vi "file control.vi"(7 "para3":u32, 8 "error in (no error)":errorcluster, 9 "op":i32, 10 "zDbName":string, 11 "para0":dbl) -> (0 "error out":errorcluster, 2 "function return":i32, 3 "para0 out":dbl, 5 "para3 out":u32)   [LabVIEW 2020, in "sqlite3.lvlib"]
uses:
  sqlite3.lvlib
  errstr.vi
  bin/sqlite3_64.dll
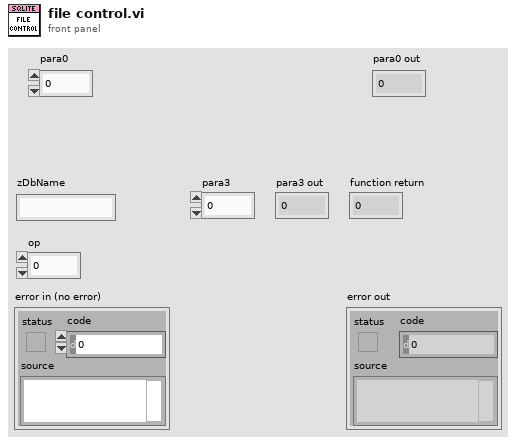
[diagram p1: front panel]
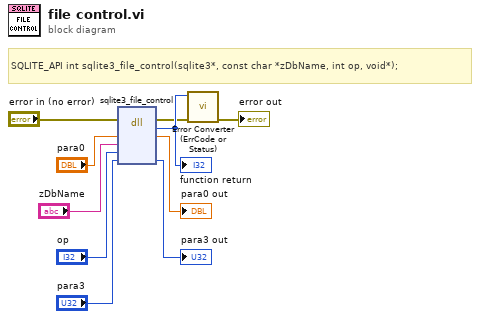
[diagram p0: block diagram]
diagram:
  # "SQLITE_API int sqlite3_file_control(sqlite3*, const char *zDbName, int op, void*);"
  n1 = dll-call lib="C:/Users/Fred.Guo/Desktop/Database-configuration/externals/sqlite3/Source/bin/sqlite3_*.*" fn="sqlite3_file_control"(error in="error in (no error)", "para0"="para0", "zDbName"="zDbName", "op"="op", "para3"="para3") -> (error out=w2:errorcluster, w10:i32, "para0"=→"para0 out":dbl, "para3"=→"para3 out":u32)  [unwired: 4 in, 1 out]
  "function return" <- w10
  n2 = call "Error Converter (ErrCode or Status).vi"("error in (no error)"=w2, "error code"=w10) -> ("error out"=→"error out":errorcluster)  [unwired: 9 in]
